vi "CheckSumGood (SubVI).vi"(11 "String in":string) -> (3 "CheckSumGood":bool)   [LabVIEW 2017, in "LV_Unicorn.lvlib"]
uses:
  LV_Unicorn.lvlib
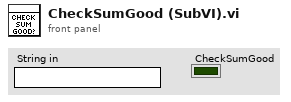
[diagram p1: front panel]
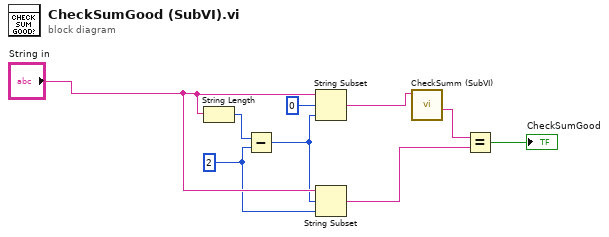
[diagram p0: block diagram]
diagram:
  w5 = 2 ("y")
  n1 = String Length(string="String in") -> (length=w2:i32)
  n2 = Subtract(x=w2, y=w5) -> (x-y=w4:i32)
  n3 = String Subset(string="String in", offset (0)=0, length (rest)=w4) -> (substring=w3:string)
  n4 = String Subset(string="String in", offset (0)=w4, length (rest)=w5) -> (substring=w8:string)
  n5 = call "CheckSumm (SubVI).vi"("Input String"=w3) -> ("CheckSumm"=w7:string)  [unwired: 7 in, 3 out]
  n6 = Equal?(x=w7, y=w8) -> (x = y?=→"CheckSumGood":bool)
